vi "6-11.vi"() -> ()   [LabVIEW 2017]
uses:
  <vilib>/Utility/file.llb/Write Delimited Spreadsheet (DBL).vi
panel:
  out "Waveform Chart":dbl(graph)
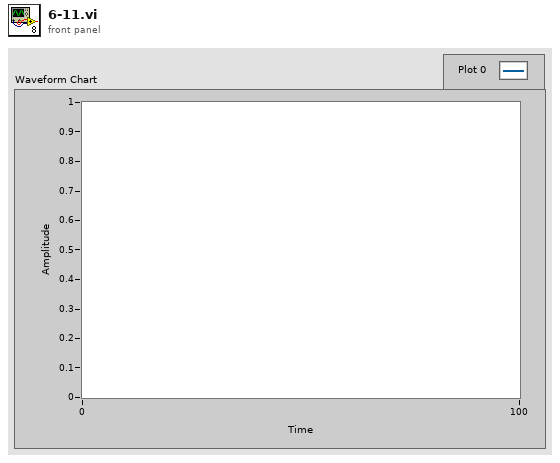
[diagram p1: front panel]
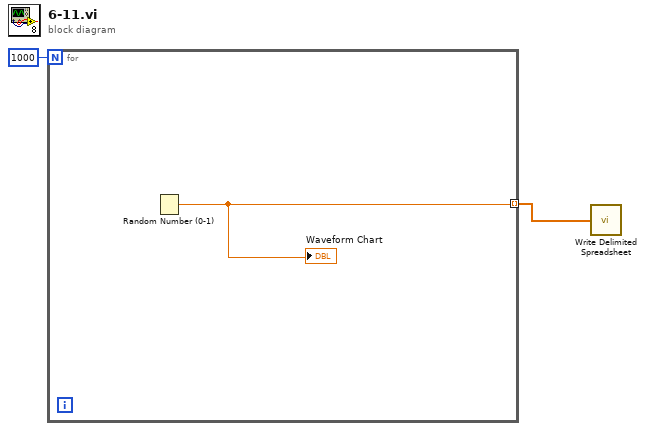
[diagram p0: block diagram]
diagram:
  n1 = for {
    N: 1000 -> [_]
    tunnel: [w3] -> w1 mode=indexing
    n2 = Random Number (0-1)() -> (number: 0 to 1=w3:dbl)
    "Waveform Chart" <- w3
  }
  n3 = call-poly <vilib>:"Write Delimited Spreadsheet.vi"("1D data"=w1) -> ()  [unwired: 13 in, 2 out]
